vi "Get_Image_Diff_Notifier.vi"() -> (3 "notifier out":refnum<notifier>)   [LabVIEW 2012]
uses:
  <vilib>/vision/Image Controls.llb/IMAQ Image.ctl
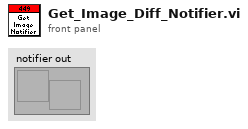
[diagram p1: front panel]
types:
  T1 = typedef "IMAQ Image.ctl" = refnum<image>
  T2 = cluster{"Image Out Light":T1, "Image Out Light":T1}
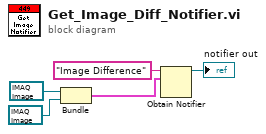
[diagram p0: block diagram]
diagram:
  n1 = Bundle("Image Out Light"=T1 refnum, "Image Out Light"=T1 refnum) -> (w3:T2)  [unwired: 1 in]
  n2 = Obtain Notifier(name (unnamed)="Image Difference", notification data type=w3) -> (notifier out=→"notifier out":refnum<notifier>)  [unwired: 2 in, 2 out]
